vi "BRig_dataTrial_Cue2_iTrial_High.vi"() -> (2 "output_Cue2_iTrial_High":i32)   [LabVIEW 2014]
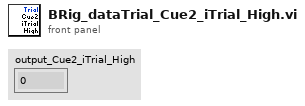
[diagram p1: front panel]
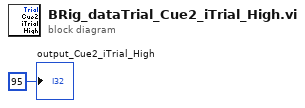
[diagram p0: block diagram]
diagram:
  "output_Cue2_iTrial_High" <- 95 ("output_iBlock")
